vi "PLC.vi"(8 "error in":errorcluster, 10 "Message Queues":T3, 11 "Notifiers":T4) -> (0 "error out":errorcluster)   [LabVIEW 2014, in "PLC.lvlib"]
uses:
  PLC.lvlib
  support/Message Queue/Message Queue.lvlib
  Model/Model.lvlib
  <vilib>/ErrorRing/Error Ring.xnode
  Logger/Logger.lvlib
  DAQ/DAQ.lvlib
  support/Global names.vi
  <vilib>/Utility/error.llb/Error Cluster From Error Code.vi
  support/Notifiers/Notifiers.ctl
  Support/Notifiers/Notifiers.lvlib
  support/Message Queue/Message Cluster.ctl
  support/Message Queue/All Message Queues.ctl
  Type definitions/PLC Data.ctl
  DAQ/TypeDefs/DAQ data.ctl
panel:
  in  "PLC Data":T1={"DAQ data"={"Power switch (DI)"={"Channel"="myDAQ2/port0/line0", "Data"=FALSE}, "Dispose barrel (DI)"={"Channel"="myDAQ2/port0/line1", "Data"=FALSE}, "Pump status (DO)"={"Channel"="myDAQ2/port0/line2", "Data"=FALSE}, "Barrel position (AI)"={"Channel"="myDAQ2/ai0", "Data"=0.0}}, "Run process"=FALSE}
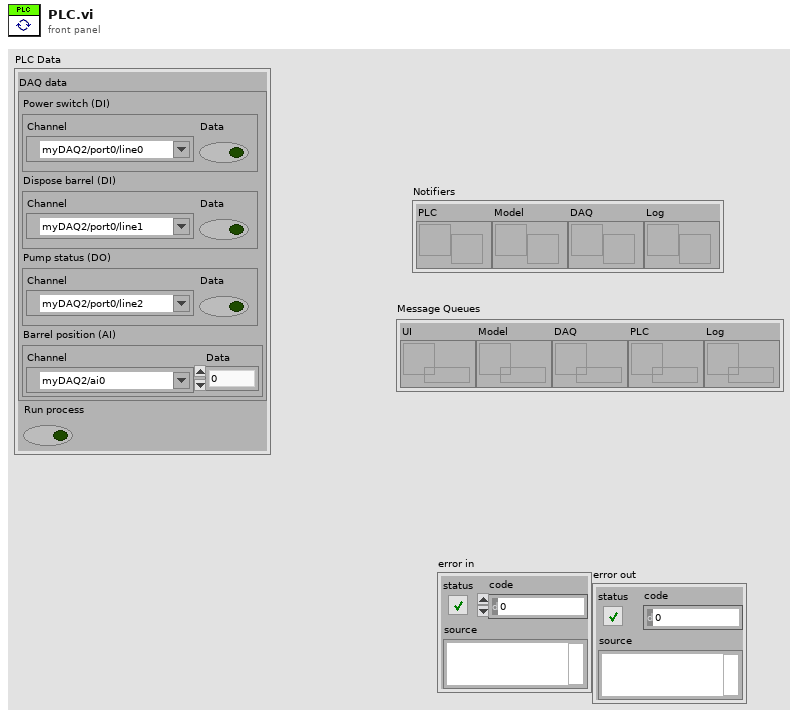
[diagram p1: front panel]
types:
  T1 = typedef "PLC.lvlib/PLC Data.ctl" = cluster{"DAQ data":T2, "Run process":bool}
  T2 = typedef "DAQ.lvlib/DAQ data.ctl" = cluster{"Power switch (DI)":cluster{"Channel":tag, "Data":bool}, "Dispose barrel (DI)":cluster{"Channel":tag, "Data":bool}, "Pump status (DO)":cluster{"Channel":tag, "Data":bool}, "Barrel position (AI)":cluster{"Channel":tag, "Data":dbl}}
  T3 = typedef "Message Queue.lvlib/All Message Queues.ctl" = cluster{"UI":refnum<queue>, "Model":refnum<queue>, "DAQ":refnum<queue>, "PLC":refnum<queue>, "Log":refnum<queue>}
  T4 = typedef "Notifiers.lvlib/Notifiers.ctl" = cluster{"PLC":refnum<notifier>, "Model":refnum<notifier>, "DAQ":refnum<notifier>, "Log":refnum<notifier>}
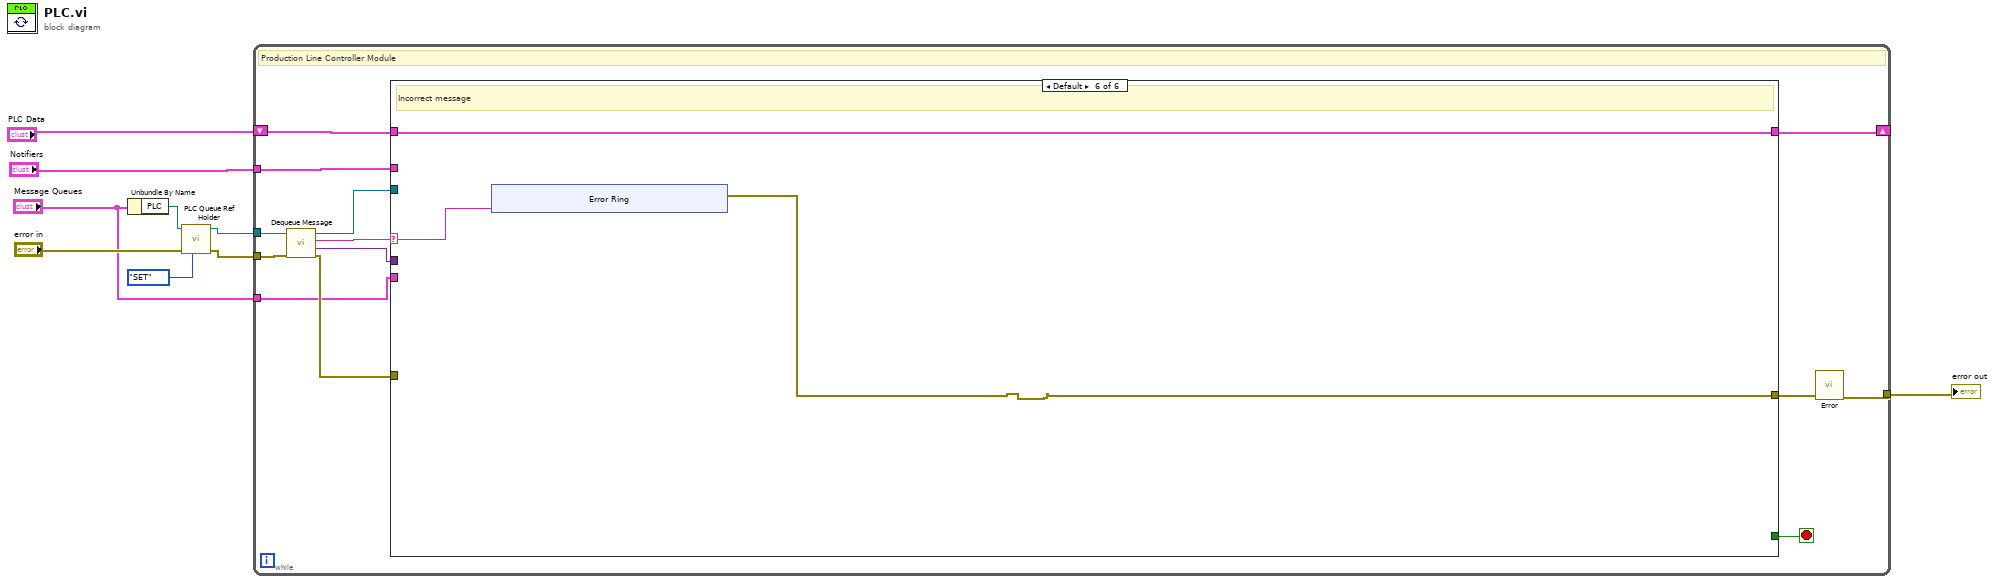
[diagram p0: block diagram]
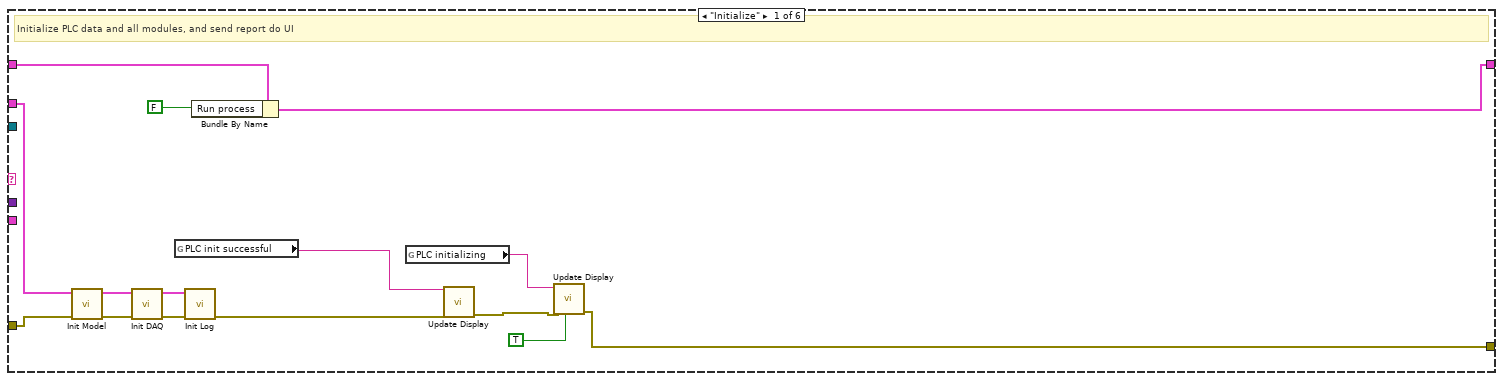
[diagram p2: hidden frame]
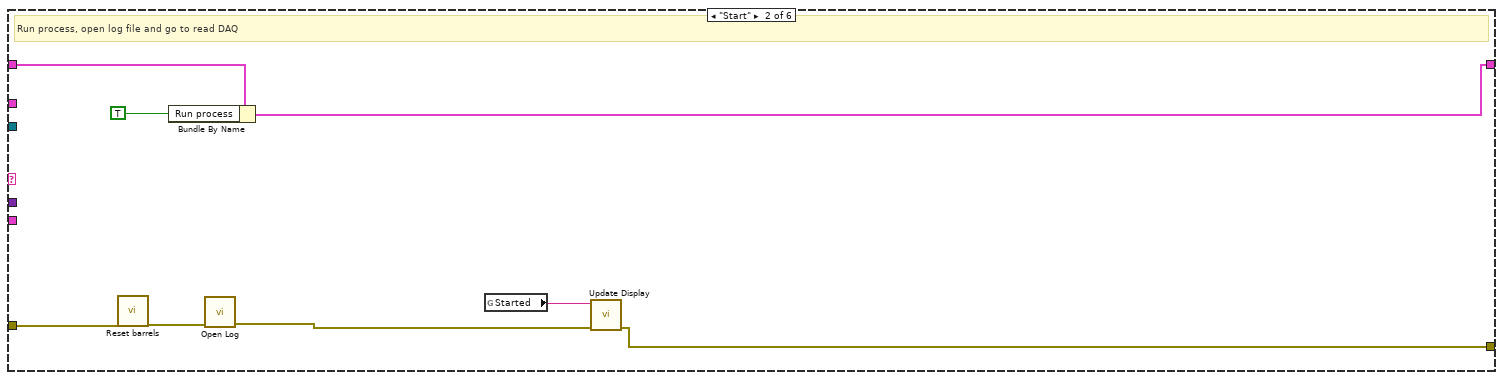
[diagram p3: hidden frame]
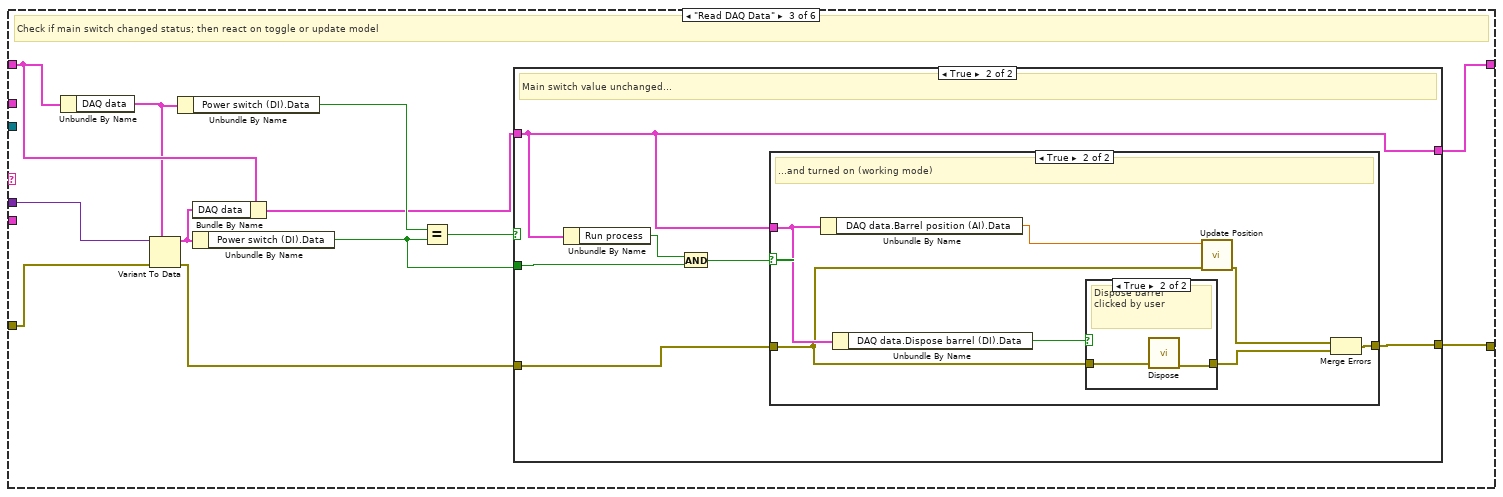
[diagram p4: hidden frame]
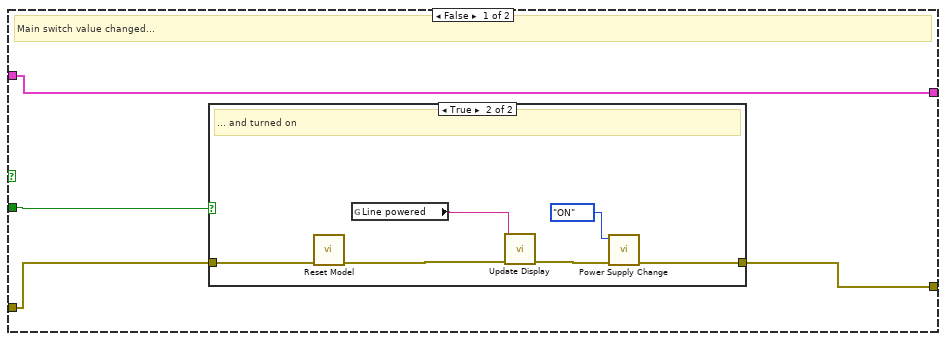
[diagram p5: hidden frame]
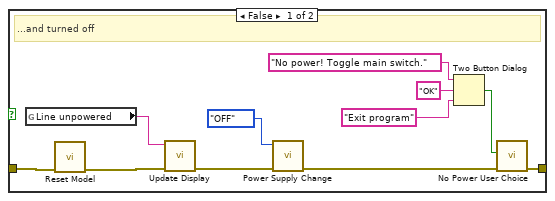
[diagram p6: hidden frame]
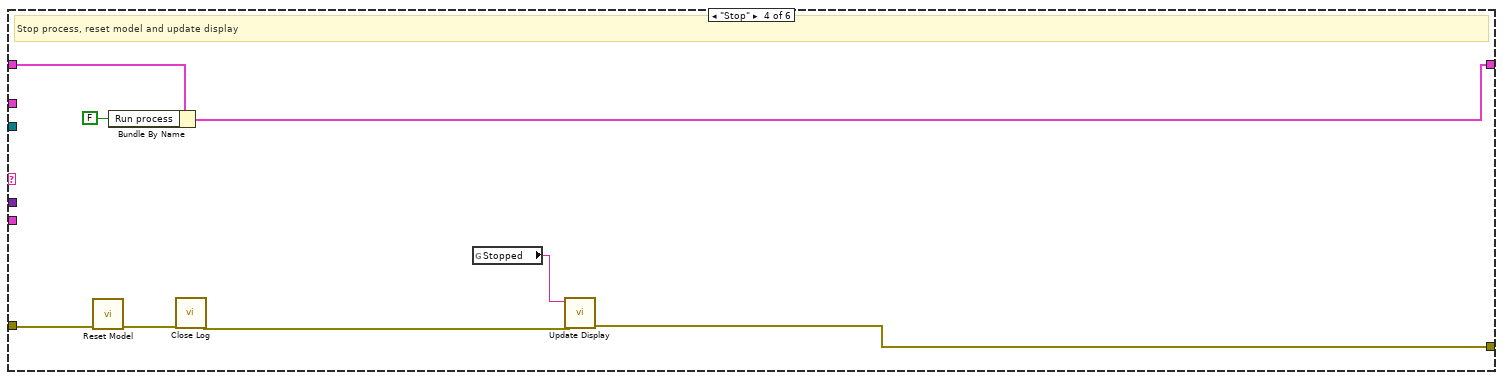
[diagram p9: hidden frame]
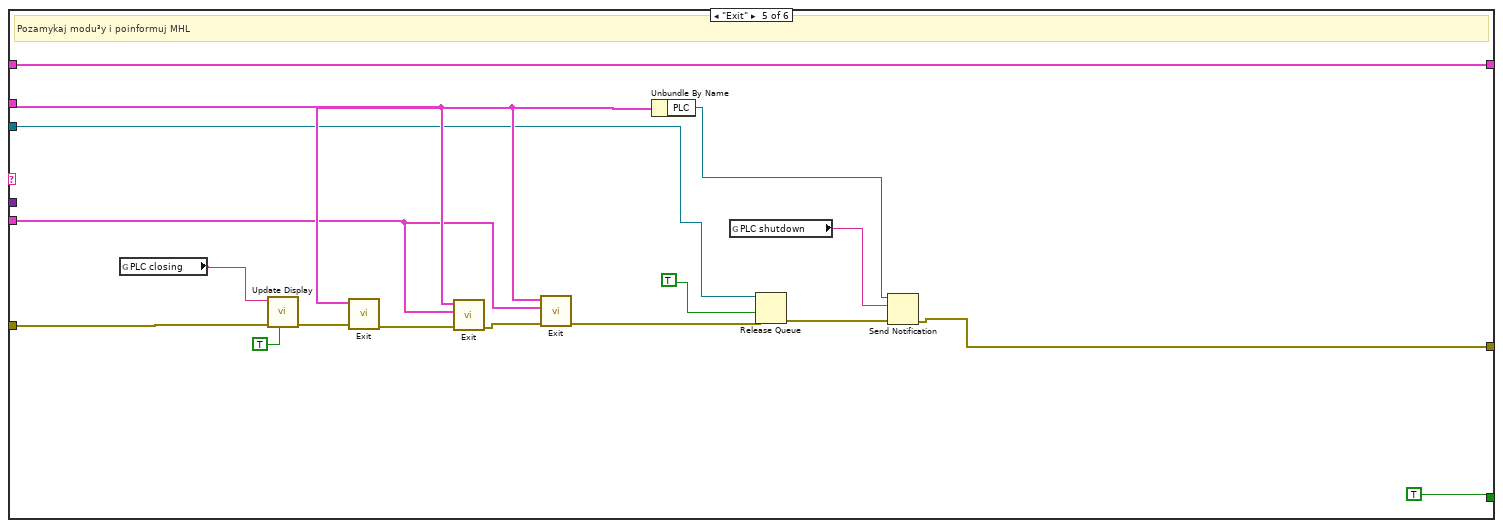
[diagram p10: hidden frame]
diagram:
  n1 = Unbundle By Name("Message Queues") -> ("PLC"=w4:refnum<queue>)
  n2 = call "PLC Queue Ref Holder.vi"("Action"=enum16{"GET", "SET"}."SET", "error in"="error in", "Message Queue In"=w4) -> ("error out"=w5:errorcluster, "Input Message Queue"=w3:refnum<queue>)  [unwired: 7 in]
  n3 = while {
    tunnel: "Notifiers" -> [w22]
    tunnel: w3 -> [w21]
    tunnel: w5 -> [w20]
    tunnel: [w11] -> w9
    tunnel: "Message Queues" -> [w17]
    shift-right: [w15] -> _
    shift-left: "PLC Data" -> [w14]
    stop <- w18 stop-if-true
    # "Production Line Controller Module"
    n4 = call "Dequeue Message.vi"("error in (no error)"=w20, "Message Queue"=w21) -> ("error out"=w19:errorcluster, "Message Data"=w16:variant, "Message"=w10:string, "dup Message Queue"=w13:refnum<queue>)  [unwired: 6 in]
    n5 = case shown="Default" w10 {
      selector: w10 -> [_ _ _ _ _ w122]
      tunnel: w22 -> [w33 _ _ _ w118 _]
      tunnel: w19 -> [w31 w40 w56 w99 w105 _]
      tunnel: w13 -> [_ _ _ _ w107 _]
      tunnel: [_ _ _ _ TRUE _] -> w18
      tunnel: [w27 w42 w46 w97 w110 w121] -> w12
      tunnel: w17 -> [_ _ _ _ w117 _]
      tunnel: w16 -> [_ _ w57 _ _ _]
      tunnel: w14 -> [w37 w45 w55 w103 w106 w123]
      tunnel: [w36 w44 w47 w101 w106 w123] -> w15
      frame "Initialize" {
        # "Initialize PLC data and all modules, and send report do UI"
        n6 = call "Init Model.vi"("error in"=w31, "Notifiers in"=w33) -> ("error out"=w30:errorcluster, "Notifiers out"=w32:T4)  [unwired: 8 in]
        n7 = call "Init DAQ.vi"("error in"=w30, "Notifiers in"=w32) -> ("error out"=w34:errorcluster, "Notifiers out"=w35:T4)  [unwired: 8 in]
        n8 = global read "Global names.vi" "PLC init successful"() -> (w25:string)
        n9 = call "Init Log.vi"("error in"=w34, "Notifiers in"=w35) -> ("error out"=w23:errorcluster)  [unwired: 8 in, 1 out]
        n10 = Bundle By Name(cluster=w37, "Run process"=FALSE) -> (w36:T1)
        n11 = global read "Global names.vi" "PLC initializing"() -> (w24:string)
        n12 = call "Update Display.vi"("error in"=w23, "Message string"=w25) -> ("error out"=w28:errorcluster)  [unwired: 9 in]
        n13 = call "Update Display.vi"("Priority Message? (F)"=TRUE, "error in"=w28, "Message string"=w24) -> ("error out"=w27:errorcluster)  [unwired: 8 in]
      }
      frame "Start" {
        # "Run process, open log file and go to read DAQ"
        n14 = call "Reset barrels.vi"("error in"=w40) -> ("error out"=w39:errorcluster)  [unwired: 10 in]
        n15 = Bundle By Name(cluster=w45, "Run process"=TRUE) -> (w44:T1)
        n16 = call "Open Log.vi"("error in"=w39) -> ("error out"=w38:errorcluster)  [unwired: 10 in]
        n17 = global read "Global names.vi" "Started"() -> (w41:string)
        n18 = call "Update Display.vi"("error in"=w38, "Message string"=w41) -> ("error out"=w42:errorcluster)  [unwired: 9 in]
      }
      frame "Read DAQ Data" {
        # "Check if main switch changed status; then react on toggle or update model"
        n19 = Unbundle By Name(w55) -> ("DAQ data"=w54:T2)
        n20 = Variant To Data(error in=w56, type=w54, Variant=w57) -> (data=w50:T2, error out=w48:errorcluster)
        n21 = Unbundle By Name(w54) -> ("Power switch (DI).Data"=w53:bool)
        n22 = Bundle By Name(cluster=w55, "DAQ data"=w50) -> (w49:T1)
        n23 = Unbundle By Name(w50) -> ("Power switch (DI).Data"=w51:bool)
        n24 = Equal?(x=w53, y=w51) -> (x = y?=w52:bool)
        n25 = case shown="True" w52 {
          tunnel: [w61 w83] -> w46
          tunnel: w51 -> [w60 w80]
          tunnel: w49 -> [w58 w79]
          tunnel: w48 -> [w59 w84]
          tunnel: [w58 w79] -> w47
          frame False {
            # "Main switch value changed..."
            n26 = case shown="True" w60 {
              tunnel: [w64 w74] -> w61
              tunnel: w59 -> [w63 w75]
              frame False {
                # "...and turned off"
                n27 = global read "Global names.vi" "Line unpowered"() -> (w62:string)
                n28 = call "Reset Model.vi"("error in"=w63) -> ("error out"=w66:errorcluster)  [unwired: 10 in]
                n29 = call "Update Display.vi"("error in"=w66, "Message string"=w62) -> ("error out"=w68:errorcluster)  [unwired: 9 in]
                n30 = call "Power Supply Change.vi"("error in"=w68, "Power status"=enum16{"OFF", "ON"}."OFF") -> ("error out"=w65:errorcluster)  [unwired: 9 in]
                n31 = Two Button Dialog(message="No power! Toggle main switch.", 1:"Exit program" ("F button name (\"Cancel\")"), 2:"OK" ("button name (\"OK\")")) -> (T button?=w69:bool)
                n32 = call "No Power User Choice.vi"("error in (no error)"=w65, "T button?"=w69) -> ("error out"=w64:errorcluster)  [unwired: 9 in]
              }
              frame True {
                # "... and turned on"
                n33 = call "Reset Model.vi"("error in"=w75) -> ("error out"=w76:errorcluster)  [unwired: 10 in]
                n34 = global read "Global names.vi" "Line powered"() -> (w73:string)
                n35 = call "Update Display.vi"("error in"=w76, "Message string"=w73) -> ("error out"=w78:errorcluster)  [unwired: 9 in]
                n36 = call "Power Supply Change.vi"("error in"=w78, "Power status"=enum16{"OFF", "ON"}."ON") -> ("error out"=w74:errorcluster)  [unwired: 9 in]
              }
            }
          }
          frame True {
            # "Main switch value unchanged..."
            n37 = Unbundle By Name(w79) -> ("Run process"=w81:bool)
            n38 = And(x=w81, y=w80) -> (x .and. y?=w82:bool)
            n39 = case shown="True" w82 {
              tunnel: w79 -> [_ w91]
              tunnel: w84 -> [w85 w90]
              tunnel: [w85 w89] -> w83
              frame False {
                # "...and turned off (idle)"
              }
              frame True {
                # "...and turned on (working mode)"
                n40 = Unbundle By Name(w91) -> ("DAQ data.Barrel position (AI).Data"=w86:dbl)
                n41 = Unbundle By Name(w91) -> ("DAQ data.Dispose barrel (DI).Data"=w92:bool)
                n42 = case shown="True" w92 {
                  tunnel: w90 -> [w93 w95]
                  tunnel: [w93 w94] -> w87
                  frame False {
                  }
                  frame True {
                    # "Dispose barrel\nclicked by user"
                    n43 = call "Dispose.vi"("error in (no error)"=w95) -> ("error out"=w94:errorcluster)  [unwired: 10 in]
                  }
                }
                n44 = call "Update Position.vi"("error in (no error)"=w90, "Position"=w86) -> ("error out"=w88:errorcluster)  [unwired: 9 in]
                n45 = Merge Errors(w88, w87) -> (w89:errorcluster)
              }
            }
          }
        }
      }
      frame "Stop" {
        # "Stop process, reset model and update display"
        n46 = call "Reset Model.vi"("error in"=w99) -> ("error out"=w98:errorcluster)  [unwired: 10 in]
        n47 = Bundle By Name(cluster=w103, "Run process"=FALSE) -> (w101:T1)
        n48 = call "Close Log.vi"("error in"=w98) -> ("error out"=w96:errorcluster)  [unwired: 10 in]
        n49 = global read "Global names.vi" "Stopped"() -> (w100:string)
        n50 = call "Update Display.vi"("error in"=w96, "Message string"=w100) -> ("error out"=w97:errorcluster)  [unwired: 9 in]
      }
      frame "Exit" {
        # "Pozamykaj modu³y i poinformuj MHL"
        n51 = global read "Global names.vi" "PLC closing"() -> (w112:string)
        n52 = call "Update Display.vi"("Priority Message? (F)"=TRUE, "error in"=w105, "Message string"=w112) -> ("error out"=w109:errorcluster)  [unwired: 8 in]
        n53 = call "Exit.vi"("error in"=w109, "Notifiers"=w118) -> ("error out"=w108:errorcluster)  [unwired: 9 in]
        n54 = call "Exit.vi"("error in"=w108, "Message Queues"=w117, "Notifiers"=w118) -> ("error out"=w113:errorcluster)  [unwired: 8 in]
        n55 = call "Exit.vi"("error in"=w113, "Message Queues"=w117, "Notifiers"=w118) -> ("error out"=w104:errorcluster)  [unwired: 8 in]
        n56 = Unbundle By Name(w118) -> ("PLC"=w115:refnum<notifier>)
        n57 = global read "Global names.vi" "PLC shutdown"() -> (w111:string)
        n58 = Release Queue(queue=w107, force destroy? (F)=TRUE, error in (no error)=w104) -> (error out=w119:errorcluster)  [unwired: 2 out]
        n59 = Send Notification(notification=w111, notifier=w115, error in (no error)=w119) -> (error out=w110:errorcluster)  [unwired: 1 out]
      }
      frame Default {
        # "Incorrect message"
        n60 = xnode "Error Ring"("parameter 0"=w122) -> ("error out"=w121:errorcluster)
      }
    }
    n61 = call "Error.vi"("error in"=w12) -> ("error out"=w11:errorcluster)  [unwired: 10 in]
  }
  "error out" <- w9
